vi "TC Parse Computer Name.vi"(8 "error in (no error)":errorcluster, 9 "AVS type":T1(ring) caption="Bridge Type", 10 "computer name":string="custardpie") -> (0 "error out":errorcluster, 1 "AVS Type":T2(ring)=enum."CF_Z_Bridge")   [LabVIEW 2013]
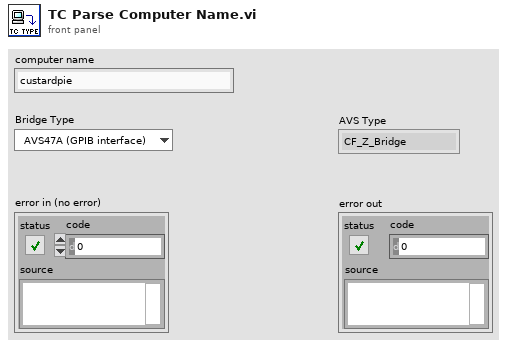
[diagram p1: front panel]
types:
  T1 = enum16{"AVS47A (GPIB interface)", "AVS47B (RS232 interface)", "AVS48", "AVS Emulation", "Impedance Bridge", "Disabled"}
  T2 = enum16{"CF", "CF_Z_Bridge", "MNK", "MNK_Z_Bridge"}
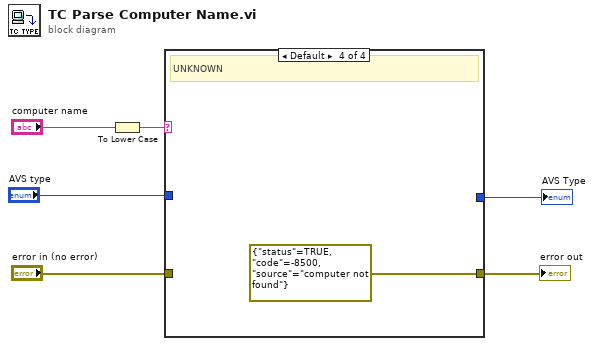
[diagram p0: block diagram]
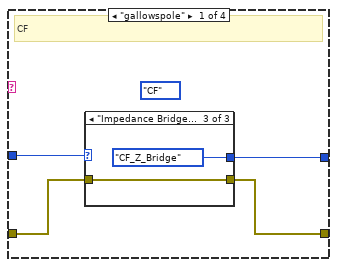
[diagram p2: hidden frame]
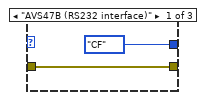
[diagram p3: hidden frame]
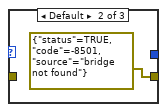
[diagram p4: hidden frame]
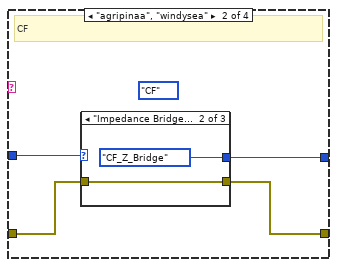
[diagram p5: hidden frame]
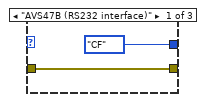
[diagram p6: hidden frame]
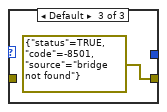
[diagram p7: hidden frame]
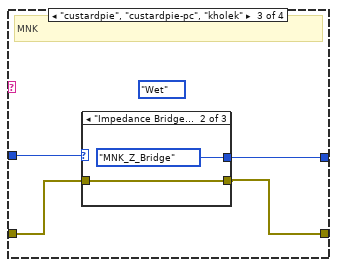
[diagram p8: hidden frame]
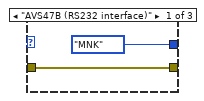
[diagram p9: hidden frame]
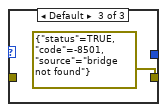
[diagram p10: hidden frame]
diagram:
  n1 = To Lower Case(string="computer name") -> (all lower case string=w1:string)
  n2 = case shown="Default" w1 {
    tunnel: "error in (no error)" -> [w7 w16 w25 _]
    tunnel: [w8 w17 w26 errorcluster {"status"=TRUE, "code"=-8500, "source"="computer not found"} ("error in (no error)")] -> w4
    tunnel: "AVS type" -> [w10 w18 w27 _]
    tunnel: [w9 w19 w28 _] -> w2
    frame "gallowspole" {
      (unwired) enum32{"CF", "Wet"}."CF" ("Type")
      # "CF"
      n3 = case shown="\"Impedance Bridge\"" w10 {
        tunnel: [T2."CF" ("AVS Type") _ T2."CF_Z_Bridge" ("AVS Type")] -> w9
        tunnel: [w11 errorcluster {"status"=TRUE, "code"=-8501, "source"="bridge not found"} ("error in (no error)") w14] -> w8
        tunnel: w7 -> [w11 _ w14]
        frame "AVS47B (RS232 interface)" {
        }
        frame Default {
        }
        frame "Impedance Bridge" {
        }
      }
    }
    frame "agripinaa", "windysea" {
      (unwired) enum32{"CF", "Wet"}."CF" ("Type")
      # "CF"
      n4 = case shown="\"Impedance Bridge\"" w18 {
        tunnel: [T2."CF" ("AVS Type") T2."CF_Z_Bridge" ("AVS Type") _] -> w19
        tunnel: [w20 w22 errorcluster {"status"=TRUE, "code"=-8501, "source"="bridge not found"} ("error in (no error)")] -> w17
        tunnel: w16 -> [w20 w22 _]
        frame "AVS47B (RS232 interface)" {
        }
        frame "Impedance Bridge" {
        }
        frame Default {
        }
      }
    }
    frame "custardpie", "custardpie-pc", "kholek" {
      (unwired) enum32{"CF", "Wet"}."Wet" ("Type")
      # "MNK"
      n5 = case shown="\"Impedance Bridge\"" w27 {
        tunnel: [T2."MNK" ("AVS Type") T2."MNK_Z_Bridge" ("AVS Type") _] -> w28
        tunnel: [w29 w31 errorcluster {"status"=TRUE, "code"=-8501, "source"="bridge not found"} ("error in (no error)")] -> w26
        tunnel: w25 -> [w29 w31 _]
        frame "AVS47B (RS232 interface)" {
        }
        frame "Impedance Bridge" {
        }
        frame Default {
        }
      }
    }
    frame Default {
      # "UNKNOWN"
    }
  }
  "error out" <- w4
  "AVS Type" <- w2
